vi "subVI_CONEX_halt.vi"(3 "Error IN":errorcluster, 5 "CONEX Cluster":T1) -> (0 "error out":errorcluster, 2 "CONEX Cluster out":T1)   [LabVIEW 2010]
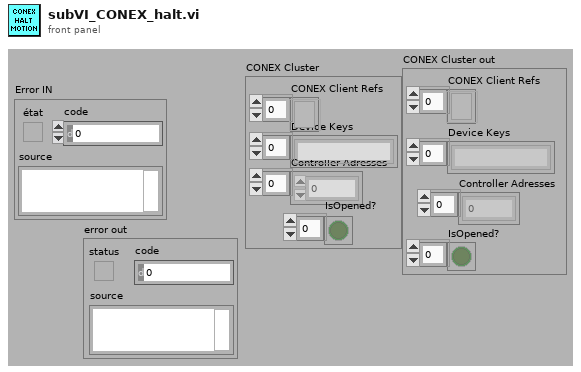
[diagram p1: front panel]
types:
  T1 = cluster{"CONEX Client Refs":refnum<k24>[], "Device Keys":string[], "Controller Adresses":i32[], "IsOpened?":bool[]}
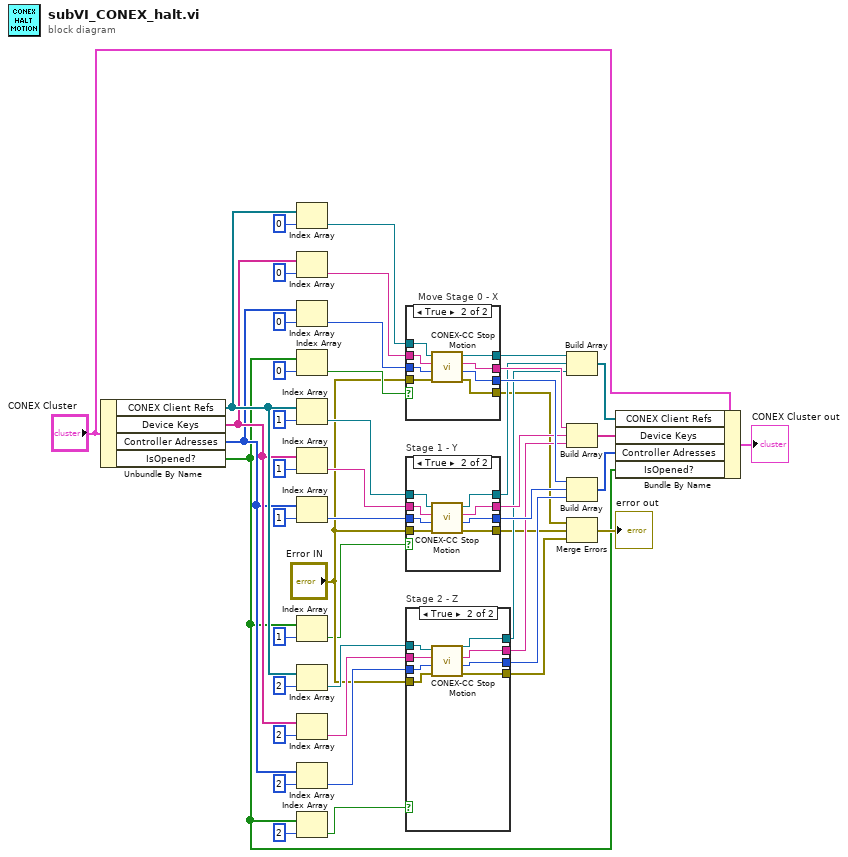
[diagram p0: block diagram]
diagram:
  n1 = Unbundle By Name("CONEX Cluster") -> ("CONEX Client Refs"=w44:refnum<k24>[], "Device Keys"=w39:string[], "Controller Adresses"=w34:i32[], "IsOpened?"=w3:bool[])
  n2 = Index Array(array=w44, index=0) -> (element=w43:refnum<k24>)
  n3 = Index Array(array=w39, index=0) -> (element=w38:string)
  n4 = Index Array(array=w34, index=0) -> (element=w33:i32)
  n5 = Index Array(array=w3, index=0) -> (element=w24:bool)
  n6 = Index Array(array=w44, index=1) -> (element=w22:refnum<k24>)
  n7 = Index Array(array=w39, index=1) -> (element=w20:string)
  n8 = Index Array(array=w34, index=1) -> (element=w17:i32)
  n9 = Index Array(array=w3, index=1) -> (element=w1:bool)
  n10 = Index Array(array=w44, index=2) -> (element=w21:refnum<k24>)
  n11 = Index Array(array=w39, index=2) -> (element=w19:string)
  n12 = Index Array(array=w34, index=2) -> (element=w18:i32)
  n13 = Index Array(array=w3, index=2) -> (element=w4:bool)
  n14 = case "Move Stage 0 - X" shown="True" w24 {
    tunnel: w43 -> [w48 w59]
    tunnel: w38 -> [w49 w58]
    tunnel: w33 -> [w50 w57]
    tunnel: "Error IN" -> [w51 w56]
    tunnel: [w48 w55] -> w32
    tunnel: [w49 w54] -> w31
    tunnel: [w50 w53] -> w30
    tunnel: [w51 w52] -> w6
    frame False {
    }
    frame True {
      n15 = call <userlib>:"CONEX-CC Stop Motion.vi"("Error IN"=w56, "Address IN"=w57, "deviceKey IN"=w58, "CONEX Client Ref IN"=w59) -> ("Error OUT"=w52:errorcluster, "Address OUT"=w53:i32, "deviceKey OUT"=w54:string, "CONEX Client Ref OUT"=w55:refnum<k24>)  [unwired: 2 in]
    }
  }
  n16 = case "Stage 1 - Y" shown="True" w1 {
    tunnel: w22 -> [w60 w71]
    tunnel: w20 -> [w61 w70]
    tunnel: w17 -> [w62 w69]
    tunnel: "Error IN" -> [w63 w68]
    tunnel: [w60 w67] -> w10
    tunnel: [w61 w66] -> w13
    tunnel: [w62 w65] -> w14
    tunnel: [w63 w64] -> w9
    frame False {
    }
    frame True {
      n17 = call <userlib>:"CONEX-CC Stop Motion.vi"("Error IN"=w68, "Address IN"=w69, "deviceKey IN"=w70, "CONEX Client Ref IN"=w71) -> ("Error OUT"=w64:errorcluster, "Address OUT"=w65:i32, "deviceKey OUT"=w66:string, "CONEX Client Ref OUT"=w67:refnum<k24>)  [unwired: 2 in]
    }
  }
  n18 = case "Stage 2 - Z" shown="True" w4 {
    tunnel: w21 -> [w72 w83]
    tunnel: w19 -> [w73 w82]
    tunnel: w18 -> [w74 w81]
    tunnel: "Error IN" -> [w75 w80]
    tunnel: [w72 w79] -> w11
    tunnel: [w73 w78] -> w12
    tunnel: [w74 w77] -> w15
    tunnel: [w75 w76] -> w8
    frame False {
    }
    frame True {
      n19 = call <userlib>:"CONEX-CC Stop Motion.vi"("Error IN"=w80, "Address IN"=w81, "deviceKey IN"=w82, "CONEX Client Ref IN"=w83) -> ("Error OUT"=w76:errorcluster, "Address OUT"=w77:i32, "deviceKey OUT"=w78:string, "CONEX Client Ref OUT"=w79:refnum<k24>)  [unwired: 2 in]
    }
  }
  n20 = Build Array(w32, w10, w11) -> (w29:refnum<k24>[])
  n21 = Build Array(w31, w13, w12) -> (w28:string[])
  n22 = Build Array(w30, w14, w15) -> (w27:i32[])
  n23 = Merge Errors(w6, w9, w8) -> (→"error out":errorcluster)
  n24 = Bundle By Name(cluster="CONEX Cluster", "CONEX Client Refs"=w29, "Device Keys"=w28, "Controller Adresses"=w27, "IsOpened?"=w3) -> (→"CONEX Cluster out":T1)
